vi "readLogStartupChecks.vi"(8 "error in (no error)":errorcluster, 10 "Parser":refnum<class "U8ArrayParserAutoIndexing.lvclass">, 11 "M1M3SAL in":refnum<class "M1M3SAL.lvclass">) -> (0 "error out":errorcluster, 2 "EventStartupChecks":variant, 3 "M1M3SAL out":refnum<class "M1M3SAL.lvclass">)   [LabVIEW 2016, in "M1M3SupportCommunicator.lvlib" / "M1M3SAL.lvclass"]
uses:
  M1M3SAL.lvclass
  Common_RT_Utilities/U8ArrayParserAutoIndexing/U8ArrayParserAutoIndexing.lvclass
  DataTypes/Topics/EventStartupChecks.ctl
  DataTypes/Topics/Parts/Timestamp.ctl
  DataTypes/Topics/M1M3SupportTopics.lvlib
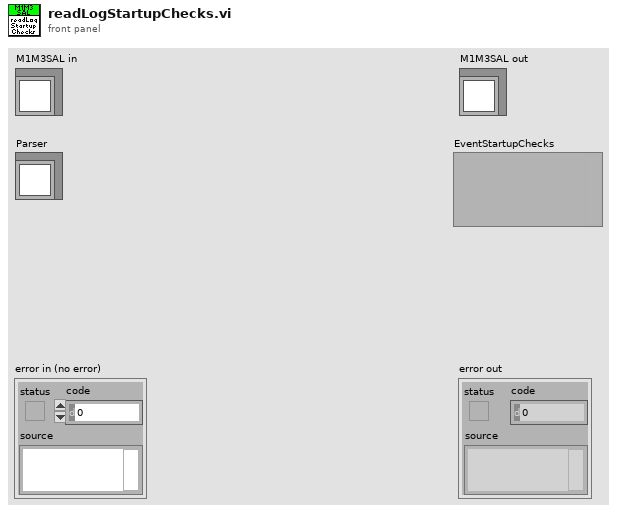
[diagram p1: front panel]
types:
  T1 = typedef "M1M3SupportTopics.lvlib/EventStartupChecks.ctl" = cluster{"Timestamp":T2, "ILCVersionsOk":bool, "DCAVersionsOk":bool, "ILCFirmwareOk":bool, "DCAFirmwareOk":bool, "ILCStatusOk":bool, "DCAStatusOk":bool}
  T2 = typedef "M1M3SupportTopics.lvlib/Timestamp.ctl" = dbl
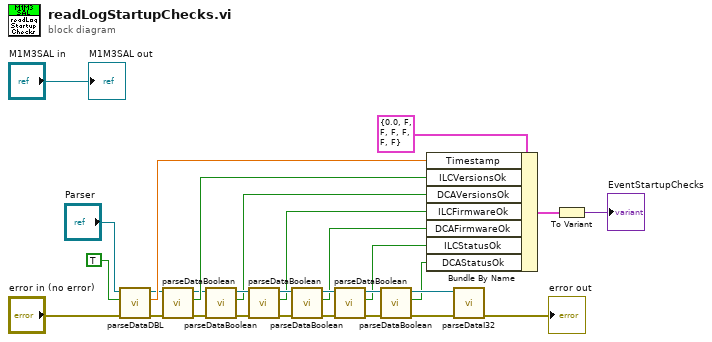
[diagram p0: block diagram]
diagram:
  n1 = call "parseDataDBL.vi"("error in (no error)"="error in (no error)", "OverrideSwapBytes"=TRUE, "U8ArrayParserAutoIndexing in"="Parser") -> ("error out"=w20:errorcluster, "Data"=w22:dbl, "U8ArrayParserAutoIndexing out"=w21:refnum<class "U8ArrayParserAutoIndexing.lvclass">)  [unwired: 6 in]
  n2 = call "parseDataBoolean.vi"("error in (no error)"=w20, "U8ArrayParserAutoIndexing in"=w21) -> ("error out"=w17:errorcluster, "Data"=w19:bool, "U8ArrayParserAutoIndexing out"=w16:refnum<class "U8ArrayParserAutoIndexing.lvclass">)  [unwired: 7 in]
  n3 = call "parseDataBoolean.vi"("error in (no error)"=w17, "U8ArrayParserAutoIndexing in"=w16) -> ("error out"=w15:errorcluster, "Data"=w5:bool, "U8ArrayParserAutoIndexing out"=w14:refnum<class "U8ArrayParserAutoIndexing.lvclass">)  [unwired: 7 in]
  n4 = call "parseDataBoolean.vi"("error in (no error)"=w15, "U8ArrayParserAutoIndexing in"=w14) -> ("error out"=w13:errorcluster, "Data"=w4:bool, "U8ArrayParserAutoIndexing out"=w12:refnum<class "U8ArrayParserAutoIndexing.lvclass">)  [unwired: 7 in]
  n5 = call "parseDataBoolean.vi"("error in (no error)"=w13, "U8ArrayParserAutoIndexing in"=w12) -> ("error out"=w11:errorcluster, "Data"=w3:bool, "U8ArrayParserAutoIndexing out"=w10:refnum<class "U8ArrayParserAutoIndexing.lvclass">)  [unwired: 7 in]
  n6 = call "parseDataBoolean.vi"("error in (no error)"=w11, "U8ArrayParserAutoIndexing in"=w10) -> ("error out"=w9:errorcluster, "Data"=w2:bool, "U8ArrayParserAutoIndexing out"=w8:refnum<class "U8ArrayParserAutoIndexing.lvclass">)  [unwired: 7 in]
  n7 = call "parseDataBoolean.vi"("error in (no error)"=w9, "U8ArrayParserAutoIndexing in"=w8) -> ("error out"=w6:errorcluster, "Data"=w1:bool, "U8ArrayParserAutoIndexing out"=w7:refnum<class "U8ArrayParserAutoIndexing.lvclass">)  [unwired: 7 in]
  n8 = Bundle By Name(cluster=T1 {"Timestamp"=0.0, "ILCVersionsOk"=FALSE, "DCAVersionsOk"=FALSE, "ILCFirmwareOk"=FALSE, "DCAFirmwareOk"=FALSE, "ILCStatusOk"=FALSE, "DCAStatusOk"=FALSE} ("EventStartupChecks"), "Timestamp"=w22, "ILCVersionsOk"=w19, "DCAVersionsOk"=w5, "ILCFirmwareOk"=w4, "DCAFirmwareOk"=w3, "ILCStatusOk"=w2, "DCAStatusOk"=w1) -> (w28:T1)
  n9 = call "parseDataI32.vi"("error in (no error)"=w6, "U8ArrayParserAutoIndexing in"=w7) -> ("error out"=→"error out":errorcluster)  [unwired: 7 in, 2 out]
  n10 = To Variant(anything=w28) -> (Variant=→"EventStartupChecks":variant)
  "M1M3SAL out" <- "M1M3SAL in"
